vi "FRCts20_Backend_Failsafe_Error.vi"(8 "error in":errorcluster) -> ()   [LabVIEW 2014, in "FRCts20_Backend_Engine.lvlib"]
uses:
  FRCts20_Backend_Engine.lvlib
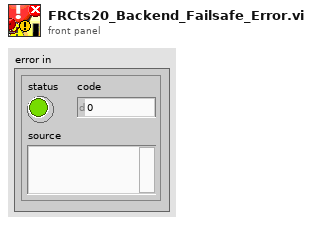
[diagram p1: front panel]
types:
  T1 = enum16{"open", "replace", "create", "open or create", "replace or create", "replace or create with confirmation"}
  T2 = enum32{"invalid app kind", "Development System", "Run Time System", "Student Edition", "Embedded LabVIEW", "Evaluation", "Custom"}
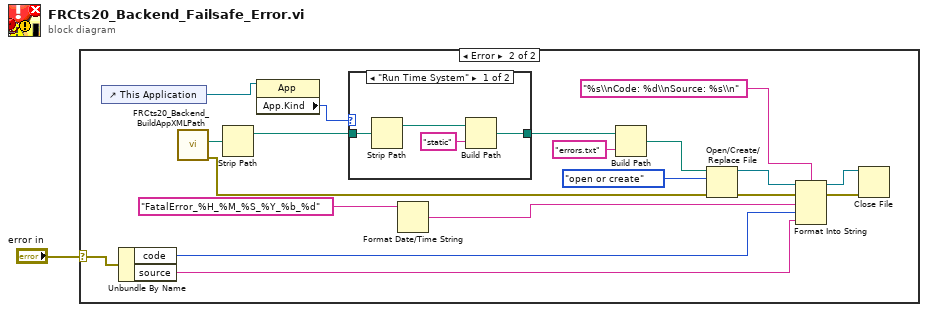
[diagram p0: block diagram]
diagram:
  n1 = case shown="Error" "error in" {
    selector: "error in" -> [_ w10]
    frame No Error {
    }
    frame Error {
      n2 = control-ref of="This Application"() -> (w5:refnum<vi>)
      n3 = Unbundle By Name(w10) -> ("code"=w8:i32, "source"=w7:string)
      n4 = call "FRCts20_Backend_BuildAppXMLPath.vi"() -> ("error out"=w12:errorcluster, "Path Out"=w11:path)  [unwired: 10 in]
      n5 = Strip Path(path=w11) -> (stripped path=w3:path)  [unwired: 1 out]
      n6 = property class="App"(reference=w5) -> ("App.Kind"=w4:T2)  [unwired: 1 in, 2 out]
      n7 = case shown="\"Run Time System\"" w4 {
        tunnel: w3 -> [w24 w25]
        tunnel: [w21 w25] -> w2
        frame "Run Time System" {
          n8 = Strip Path(path=w24) -> (stripped path=w23:path)  [unwired: 1 out]
          n9 = Build Path(base path=w23, name or relative path="static") -> (appended path=w21:path)
        }
        frame "Development System", Default {
        }
      }
      n10 = Format Date/Time String(time format string (%c)="FatalError_%H_%M_%S_%Y_%b_%d") -> (date/time string=w9:string)  [unwired: 2 in]
      n11 = Build Path(base path=w2, name or relative path="errors.txt") -> (appended path=w15:path)
      n12 = Open/Create/Replace File(file path (use dialog)=w15, error in=w12, operation (0:open)=T1."open or create") -> (refnum out=w20:refnum<file>, error out=w19:errorcluster)  [unwired: 3 in, 1 out]
      n13 = Format Into String(format string="%s\\nCode: %d\\nSource: %s\\n", initial string=w20, error in=w19, w9, w8, w7) -> (resulting string=w18:refnum<file>, error out=w17:errorcluster)
      n14 = Close File(refnum=w18, error in=w17) -> ()  [unwired: 2 out]
    }
  }
